vi "Digitizer to Amp.vi"(10 "DAQdata":i16[](array[numeric]), 11 "fullscale":dbl) -> (3 "A":dbl)   [LabVIEW 2021]
uses:
  <vilib>/measure/mascope.llb/Amplitude and Levels 1 chan.vi
  <vilib>/measure/NI_MAPro.lvlib
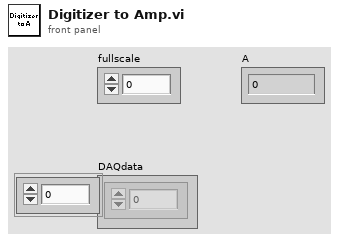
[diagram p1: front panel]
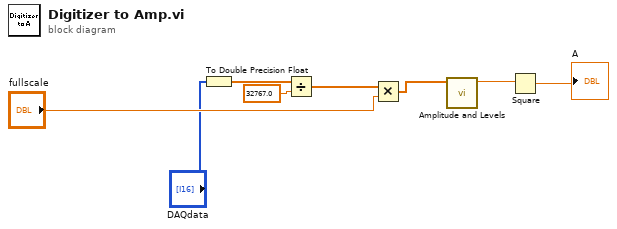
[diagram p0: block diagram]
diagram:
  n1 = To Double Precision Float(number="DAQdata") -> (double precision float=w6:dbl[])
  n2 = Divide(x=w6, y=32767.0) -> (x/y=w7:dbl[])
  n3 = Multiply(x=w7, y="fullscale") -> (x*y=w3:dbl[])
  n4 = call-poly <vilib>:"Amplitude and Levels.vi"("signal in"=w3) -> ("amplitude"=w2:dbl)  [unwired: 7 in, 3 out]
  n5 = Square(x=w2) -> (x^2=→"A":dbl)
